vi "Write Fill.vi"(8 "error in (no error)":errorcluster, 10 "Fill":bool, 11 "Rectangle in":refnum<class "Rectangle.lvclass">=refnum) -> (0 "error out":errorcluster, 3 "Rectangle out":refnum<class "Rectangle.lvclass">)   [LabVIEW 2020]
uses:
  Rectangle.lvclass
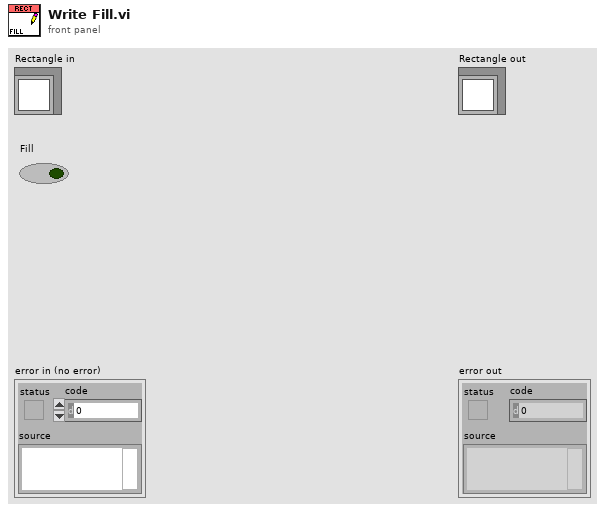
[diagram p1: front panel]
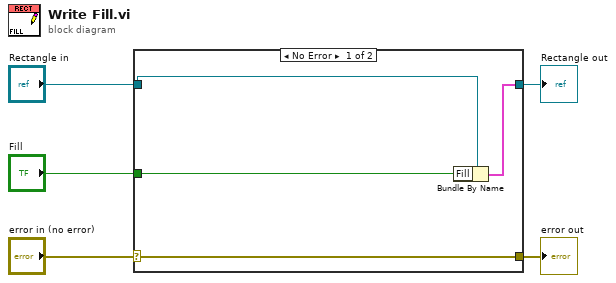
[diagram p0: block diagram]
diagram:
  n1 = case shown="No Error" "error in (no error)" {
    selector: "error in (no error)" -> [w9 w10]
    tunnel: [w9 w10] -> w4
    tunnel: [w7 w11] -> w2
    tunnel: "Rectangle in" -> [w8 w11]
    tunnel: "Fill" -> [w6 _]
    frame No Error {
      n2 = Bundle By Name(cluster=w8, "Fill"=w6) -> (w7:cluster{})
    }
    frame Error {
    }
  }
  "error out" <- w4
  "Rectangle out" <- w2
